vi "Write Transfer.vi"(8 "error in (no error)":errorcluster, 9 "transfer values":T1, 10 "id":string, 11 "Configuration Session in":refnum<class "Configuration Session.lvclass">) -> (0 "error out":errorcluster, 3 "Configuration Session out":refnum<class "Configuration Session.lvclass">, 4 "replaced?":bool)   [LabVIEW 2017, in "DSF Core.lvlib" / "Configuration Session.lvclass"]
doc: "Writes a value to a key in a specified section of the configuration data identified by <B>dsf refnum</B>. This VI modifies data in memory. To write data to disk, use the Close Config Data VI. Wire data to the <B>value</B> input to determine the polymorphic instance to use or manually select the instance."
uses:
  Configuration Session.lvclass
  Typedefs/DSF Transfer Info.ctl
  Typedefs/DSF Byte Order.ctl
  DSF Core.lvlib
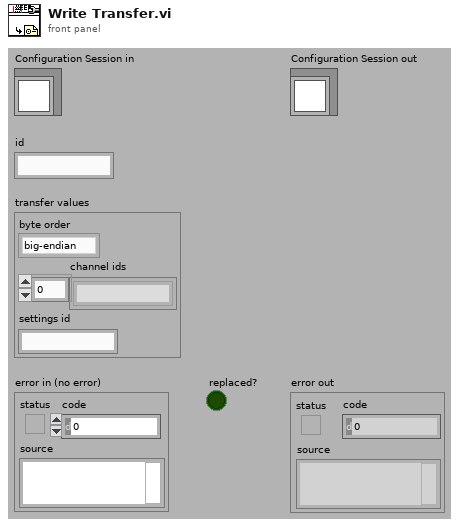
[diagram p1: front panel]
types:
  T1 = typedef "DSF Core.lvlib/DSF Transfer Info.ctl" = cluster{"byte order":T2, "channel ids":string[], "settings id":string}
  T2 = typedef "DSF Core.lvlib/DSF Byte Order.ctl" = enum8{"big-endian", "little-endian"}
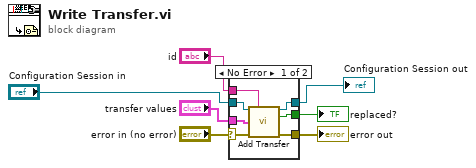
[diagram p0: block diagram]
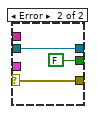
[diagram p2: hidden frame]
diagram:
  n1 = case shown="No Error" "error in (no error)" {
    selector: "error in (no error)" -> [w11 w17]
    tunnel: [w12 w17] -> w6
    tunnel: "id" -> [w14 _]
    tunnel: [w13 FALSE ("key exists?")] -> w4
    tunnel: "Configuration Session in" -> [w10 w15]
    tunnel: [w9 w15] -> w1
    tunnel: "transfer values" -> [w8 _]
    frame No Error {
      n2 = call "Add Transfer.vi"("Configuration Session in"=w10, "id"=w14, "values"=w8, "error in (no error)"=w11) -> ("Configuration Session out"=w9:refnum<class "Configuration Session.lvclass">, "plugin exists?"=w13:bool, "error out"=w12:errorcluster)  [unwired: 9 in]
    }
    frame Error {
    }
  }
  "error out" <- w6
  "replaced?" <- w4
  "Configuration Session out" <- w1
